vi "HFR500 Range Strings.vi"(5 "ppm Range":T1) -> (1 "Range Digit":string, 2 "Range String":string)   [LabVIEW 2020]
uses:
  HFR500 ppm Range.ctl
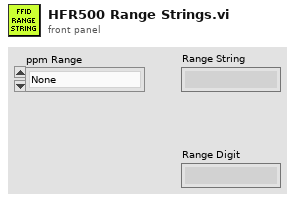
[diagram p1: front panel]
types:
  T1 = typedef "HFR500 ppm Range.ctl" = enum16{"None", "1,000", "2,000", "5,000", "10,000", "20,000", "50,000", "100,000", "200,000"}
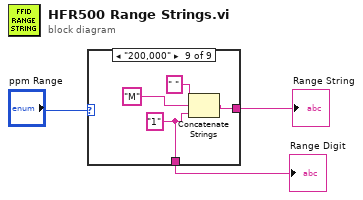
[diagram p0: block diagram]
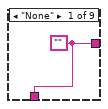
[diagram p2: hidden frame]
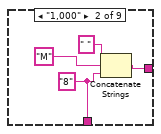
[diagram p3: hidden frame]
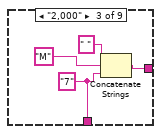
[diagram p4: hidden frame]
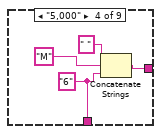
[diagram p5: hidden frame]
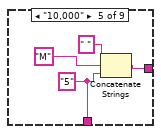
[diagram p6: hidden frame]
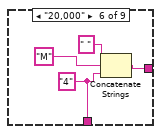
[diagram p7: hidden frame]
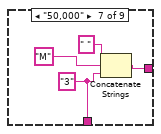
[diagram p8: hidden frame]
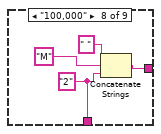
[diagram p9: hidden frame]
diagram:
  n1 = case shown="\"200,000\"" "ppm Range" {
    tunnel: [w4 w6 w10 w14 w18 w22 w26 w30 w34] -> w2
    tunnel: [w4 w5 w9 w13 w17 w21 w25 w29 w33] -> w3
    frame "None" {
      w4 = ""
    }
    frame "1,000" {
      w5 = "8"
      n2 = Concatenate Strings(" ", "M" ("string"), w5) -> (w6:string)
    }
    frame "2,000" {
      w9 = "7"
      n3 = Concatenate Strings(" ", "M" ("string"), w9) -> (w10:string)
    }
    frame "5,000" {
      w13 = "6"
      n4 = Concatenate Strings(" ", "M" ("string"), w13) -> (w14:string)
    }
    frame "10,000" {
      w17 = "5"
      n5 = Concatenate Strings(" ", "M" ("string"), w17) -> (w18:string)
    }
    frame "20,000" {
      w21 = "4"
      n6 = Concatenate Strings(" ", "M" ("string"), w21) -> (w22:string)
    }
    frame "50,000" {
      w25 = "3"
      n7 = Concatenate Strings(" ", "M" ("string"), w25) -> (w26:string)
    }
    frame "100,000" {
      w29 = "2"
      n8 = Concatenate Strings(" ", "M" ("string"), w29) -> (w30:string)
    }
    frame "200,000" {
      w33 = "1"
      n9 = Concatenate Strings(" ", "M" ("string"), w33) -> (w34:string)
    }
  }
  "Range String" <- w2
  "Range Digit" <- w3
